vi "Send UNREGISTER.vi"(8 "error in (no error)":errorcluster, 9 "Unregister Request":T1, 10 "Message loop data (in)":T2, 11 "WAMP Client in":refnum<class "WAMP Client.lvclass">) -> (0 "error out":errorcluster, 2 "Message loop data (out)":T2, 3 "WAMP Client out":refnum<class "WAMP Client.lvclass">)   [LabVIEW 2020, in "wamplv.lvlib" / "WAMP Client.lvclass"]
uses:
  <vilib>/samangh/wamplv/WAMP Client/WAMP Client.lvclass
  <vilib>/samangh/wamplv/WAMP Client/TypeDef/Message Loop Shift Reg Data.ctl
  <vilib>/samangh/wamplv/WAMP Client/TypeDef/REGISTER Request Data.ctl
  <vilib>/samangh/wamplv/WAMP Client/TypeDef/Success or error.ctl
  <vilib>/samangh/wamplv/WAMP Client/TypeDef/Combined error.ctl
  <vilib>/samangh/wamplv/WAMP Client/TypeDef/WAMP Error Payload.ctl
  <vilib>/samangh/wamplv/WAMP Client/TypeDef/INVOCATION payload.ctl
  <vilib>/samangh/wamplv/WAMP Client/TypeDef/Publish Requests Map.ctl
  <vilib>/samangh/wamplv/WAMP Client/TypeDef/PUBLISH Request Data.ctl
  <vilib>/samangh/wamplv/WAMP Client/TypeDef/PUBLISH Result.ctl
  <vilib>/samangh/wamplv/WAMP Client/TypeDef/Endpoint Data.ctl
  <vilib>/samangh/wamplv/WAMP Client/TypeDef/CALL Request Map.ctl
  <vilib>/samangh/wamplv/WAMP Client/TypeDef/CALL Request Data.ctl
  <vilib>/samangh/wamplv/WAMP Client/TypeDef/RESULT Payload.ctl
  <vilib>/samangh/wamplv/WAMP Client/TypeDef/SUBSCRIBE Requests Map.ctl
  <vilib>/samangh/wamplv/WAMP Client/TypeDef/SUBSCRIBE Request Data.ctl
  <vilib>/samangh/wamplv/WAMP Client/TypeDef/Subscribe Result.ctl
  <vilib>/samangh/wamplv/WAMP Client/TypeDef/Event Payload.ctl
  <vilib>/samangh/wamplv/WAMP Client/TypeDef/Subscriptions Map.ctl
  <vilib>/samangh/wamplv/WAMP Client/TypeDef/Subscription Details.ctl
  <vilib>/samangh/wamplv/WAMP Client/TypeDef/Unsubscribe Requests Map.ctl
  <vilib>/samangh/wamplv/WAMP Client/TypeDef/UNSUBSCRIBE Request Data.ctl
  <vilib>/samangh/wamplv/WAMP Client/TypeDef/UNSUBSCRIBE Result.ctl
  <vilib>/samangh/wamplv/WAMP Client/TypeDef/Unregister requests map.ctl
  <vilib>/samangh/wamplv/WAMP Client/TypeDef/Unregister request.ctl
  <vilib>/samangh/wamplv/WAMP Message Codes.ctl
  <vilib>/samangh/wamplv/WAMP Client/WAMP Client.lvclass/WAMP Client.ctl
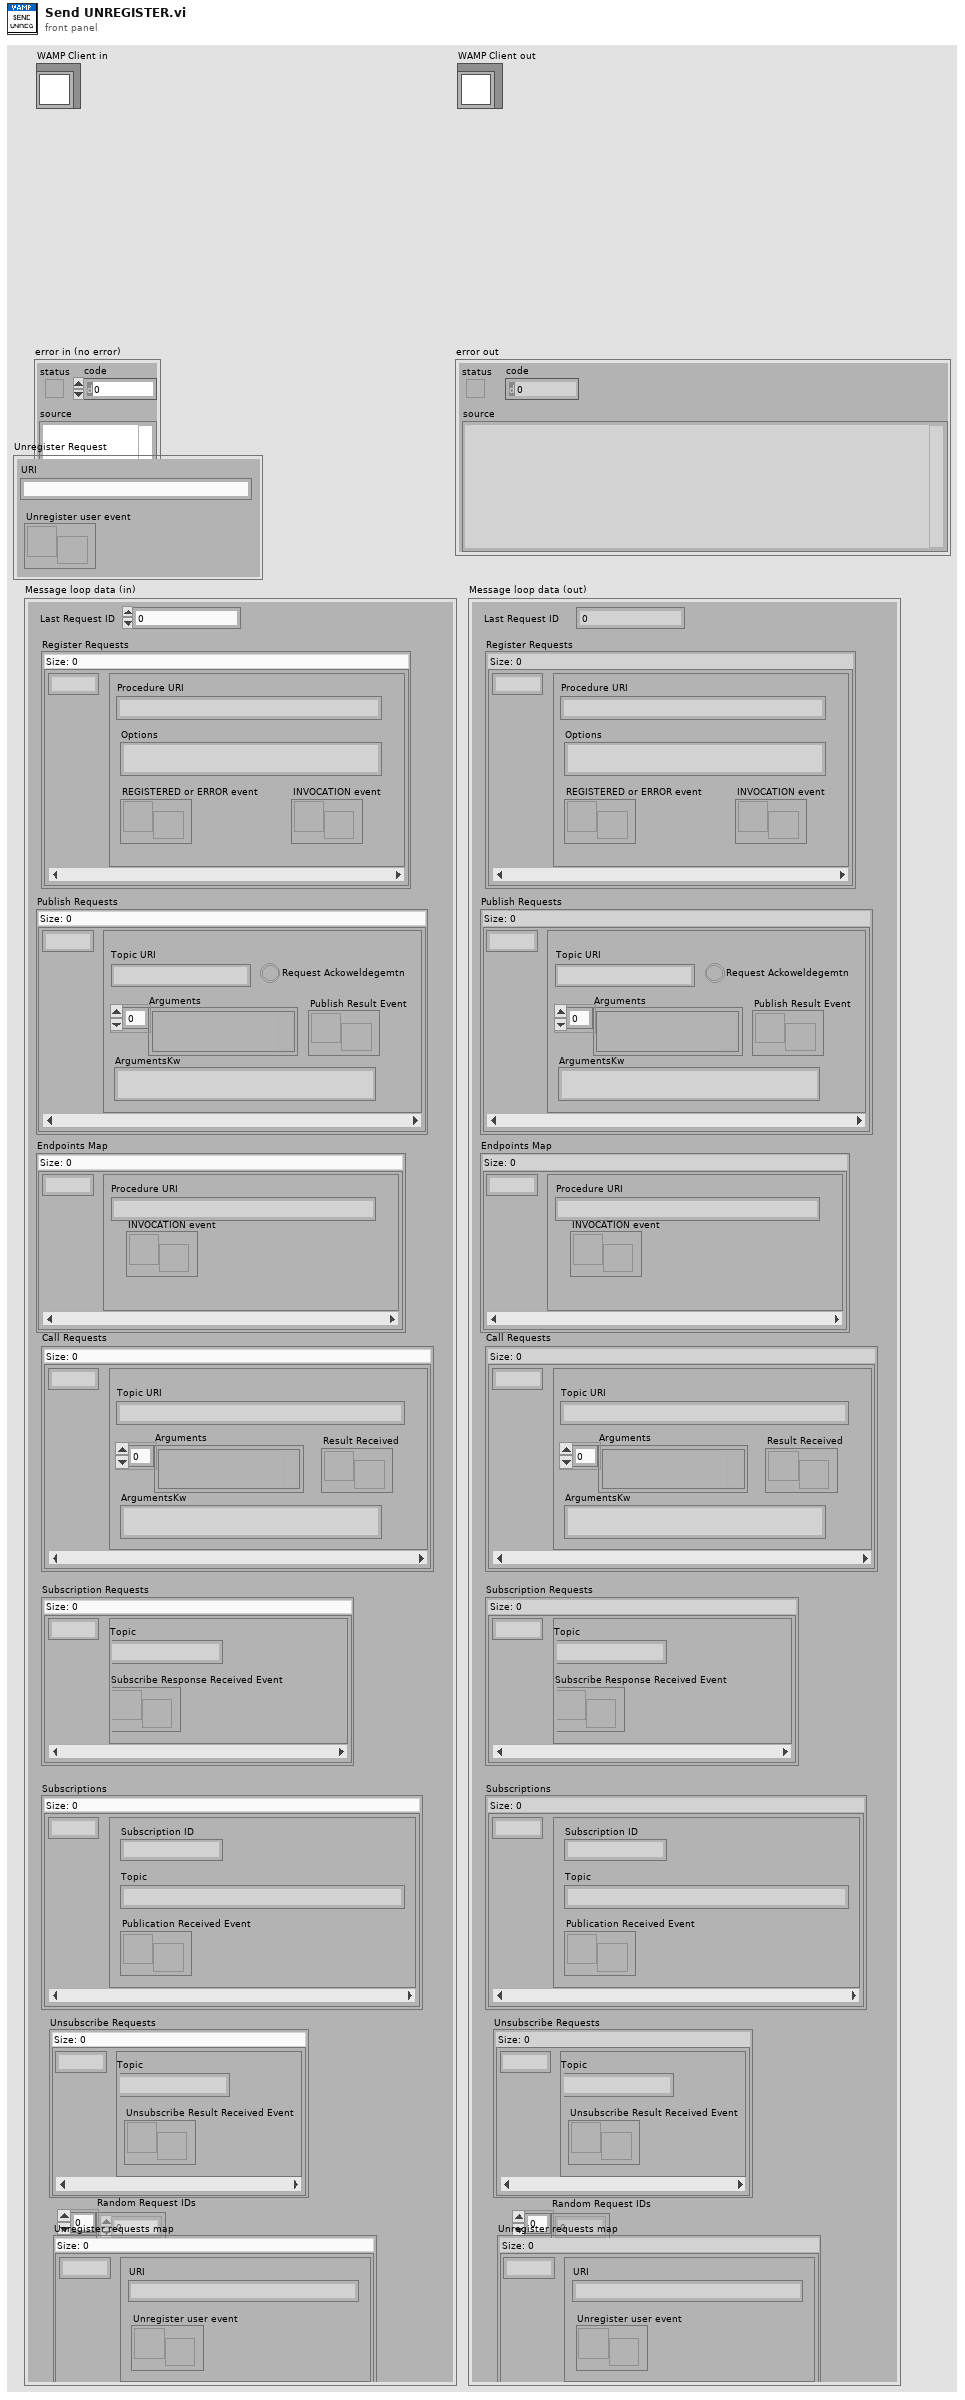
[diagram p1: front panel]
types:
  T1 = typedef "wamplv.lvlib/WAMP Client.lvclass/Unregister request.ctl" = cluster{"URI":string, "Unregister user event":refnum<user-event>}
  T2 = typedef "wamplv.lvlib/WAMP Client.lvclass/Message Loop Shift Reg Data.ctl" = cluster{"Last Request ID":u64, "Register Requests":map{u64, T3}, "Publish Requests":T4, "Endpoints Map":map{u64, T6}, "Call Requests":T7, "Subscription Requests":T9, "Subscriptions":T11, "Unsubscribe Requests":T13, "Random Request IDs":u64[], "Unregister requests map":T15}
  T3 = typedef "wamplv.lvlib/WAMP Client.lvclass/REGISTER Request Data.ctl" = cluster{"Procedure URI":string, "Options":string, "REGISTERED or ERROR event":refnum<user-event>, "INVOCATION event":refnum<user-event>}
  T4 = typedef "wamplv.lvlib/WAMP Client.lvclass/Publish Requests Map.ctl" = map{u64, T5}
  T5 = typedef "wamplv.lvlib/WAMP Client.lvclass/PUBLISH Request Data.ctl" = cluster{"Topic URI":string, "Arguments":variant[], "ArgumentsKw":string, "Publish Result Event":refnum<user-event>, "Request Ackoweldegemtn":bool}
  T6 = typedef "wamplv.lvlib/WAMP Client.lvclass/Endpoint Data.ctl" = cluster{"Procedure URI":string, "INVOCATION event":refnum<user-event>}
  T7 = typedef "wamplv.lvlib/WAMP Client.lvclass/CALL Request Map.ctl" = map{u64, T8}
  T8 = typedef "wamplv.lvlib/WAMP Client.lvclass/CALL Request Data.ctl" = cluster{"Topic URI":string, "Arguments":variant[], "ArgumentsKw":string, "Result Received":refnum<user-event>}
  T9 = typedef "wamplv.lvlib/WAMP Client.lvclass/SUBSCRIBE Requests Map.ctl" = map{u64, T10}
  T10 = typedef "wamplv.lvlib/WAMP Client.lvclass/SUBSCRIBE Request Data.ctl" = cluster{"Topic":string, "Subscribe Response Received Event":refnum<user-event>}
  T11 = typedef "wamplv.lvlib/WAMP Client.lvclass/Subscriptions Map.ctl" = map{u64, T12}
  T12 = typedef "wamplv.lvlib/WAMP Client.lvclass/Subscription Details.ctl" = cluster{"Subscription ID":u64, "Topic":string, "Publication Received Event":refnum<user-event>}
  T13 = typedef "wamplv.lvlib/WAMP Client.lvclass/Unsubscribe Requests Map.ctl" = map{u64, T14}
  T14 = typedef "wamplv.lvlib/WAMP Client.lvclass/UNSUBSCRIBE Request Data.ctl" = cluster{"Topic":string, "Unsubscribe Result Received Event":refnum<user-event>}
  T15 = typedef "wamplv.lvlib/WAMP Client.lvclass/Unregister requests map.ctl" = map{u64, T1}
  T16 = typedef "wamplv.lvlib/WAMP Client.lvclass/WAMP Message Codes.ctl" = u16
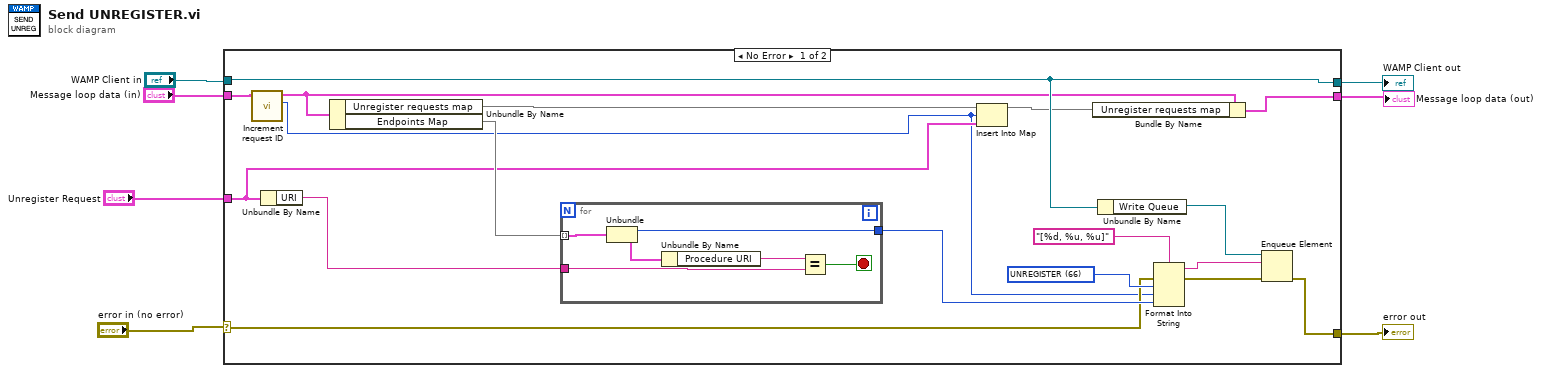
[diagram p0: block diagram]
diagram:
  n1 = case shown="No Error" "error in (no error)" {
    selector: "error in (no error)" -> [w17 w34]
    tunnel: [w20 w34] -> w6
    tunnel: [w21 w33] -> w4
    tunnel: "WAMP Client in" -> [w21 w33]
    tunnel: "Unregister Request" -> [w10 _]
    tunnel: "Message loop data (in)" -> [w14 w32]
    tunnel: [w15 w32] -> w2
    frame No Error {
      w22 = T16 66 items=["HELLO"=1, "WELCOME"=2, "ABORT"=3, "GOODBYE"=6, "ERROR"=8, "PUBLISH"=16, "PUBLISHED"=17, "SUBSCRIBE"=32, "SUBSCRIBED"=33, "UNSUBSCRIBE"=34, "UNSUBSCRIBED"=35, "EVENT"=36, "CALL"=48, "RESULT"=59, "REGISTER"=64, "REGISTERED"=65, "UNREGISTER"=66, "UNREGISTERED"=67, "INVOCATION"=68, "YIELD"=70] ("Message Codes")
      n2 = call <vilib>:"Increment request ID.vi"("Message Loop Shift Register Data (in)"=w14) -> ("New Request ID"=w8:u64, "Message Loop Shift Register Data (out)"=w9:T2)  [unwired: 9 in]
      n3 = Unbundle By Name(w10) -> ("URI"=w12:string)
      n4 = Unbundle By Name(w9) -> ("Unregister requests map"=w11:T15, "Endpoints Map"=w13:map{u64, T6})
      n5 = for {
        tunnel: [w29] -> w18
        tunnel: w13 -> [w27] mode=indexing
        tunnel: w12 -> [w26]
        stop <- w30 stop-if-true
        n6 = Unbundle(w27) -> ("key"=w29:u64, "Endpoint Data"=w31:T6)
        n7 = Unbundle By Name(w31) -> ("Procedure URI"=w28:string)
        n8 = Equal?(x=w28, y=w26) -> (x = y?=w30:bool)
      }
      n9 = Insert Into Map(map in=w11, key=w8, value=w10) -> (map out=w16:T15)  [unwired: 2 out]
      n10 = Bundle By Name(cluster=w9, "Unregister requests map"=w16) -> (w15:T2)
      n11 = Unbundle By Name(w21) -> ("Write Queue"=w19:refnum<queue>)
      n12 = Format Into String(format string="[%d, %u, %u]" ("element"), error in=w17, w22, w8, w18) -> (resulting string=w24:string, error out=w25:errorcluster)  [unwired: 1 in]
      n13 = Enqueue Element(queue=w19, element=w24, error in (no error)=w25) -> (error out=w20:errorcluster)  [unwired: 1 in, 2 out]
    }
    frame Error {
    }
  }
  "error out" <- w6
  "WAMP Client out" <- w4
  "Message loop data (out)" <- w2
